vi "BuildMaun.vi"(8 "error in (no error)":errorcluster, 10 "menu reference":refnum<k9>, 11 "PLC_Module in":refnum<class "PLC_Module.lvclass">) -> (0 "error out":errorcluster, 3 "PLC_Module out":refnum<class "PLC_Module.lvclass">)   [LabVIEW 2025, in "PLC_Module.lvlib" / "PLC_Module.lvclass"]
uses:
  PLC_Module.lvclass
  PLC_Module.lvclass/PLC_Module.ctl
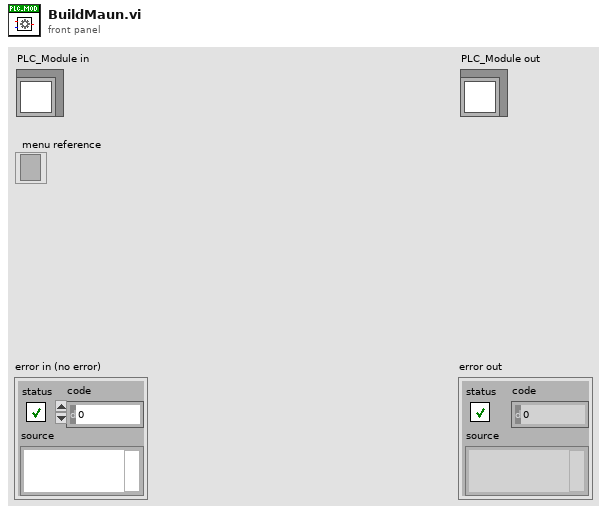
[diagram p1: front panel]
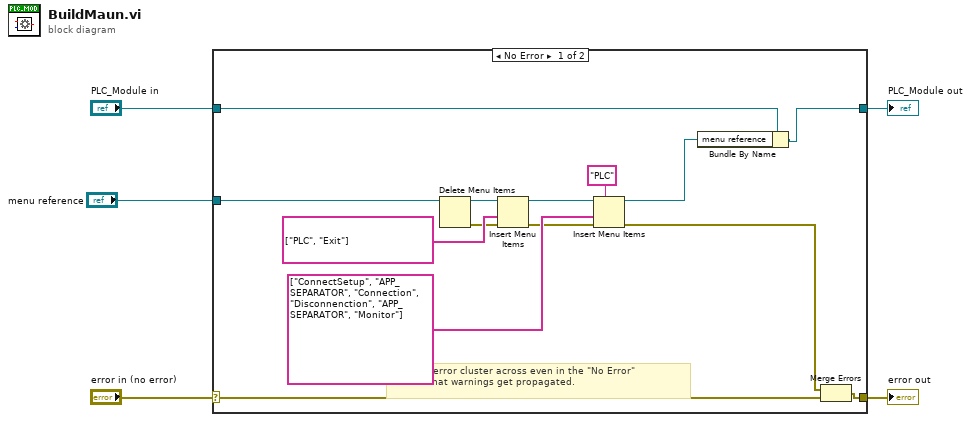
[diagram p0: block diagram]
diagram:
  n1 = case shown="No Error" "error in (no error)" {
    selector: "error in (no error)" -> [w19 w21]
    tunnel: [w13 w21] -> w4
    tunnel: [w6 w20] -> w2
    tunnel: "PLC_Module in" -> [w8 w20]
    tunnel: "menu reference" -> [w11 _]
    frame No Error {
      # "Wire the error cluster across even in the \"No Error\"\ncase so that warnings get propagated."
      n2 = Delete Menu Items(9:w11) -> (0:w9:errorcluster, 3:w10:refnum<k9>)  [unwired: 3 in]
      n3 = Insert Menu Items(6:w9, 7:string[] ["PLC", "Exit"] ("item tags"), 9:w10) -> (0:w14:errorcluster, 3:w17:refnum<k9>)  [unwired: 3 in, 1 out]
      n4 = Insert Menu Items(5:"PLC", 6:w14, 7:string[] ["ConnectSetup", "APP_SEPARATOR", "Connection", "Disconnenction", "APP_SEPARATOR", "Monitor"] ("item tags"), 9:w17) -> (0:w12:errorcluster, 3:w7:refnum<k9>)  [unwired: 2 in, 1 out]
      n5 = Bundle By Name(cluster=w8, "menu reference"=w7) -> (w6:refnum<class "PLC_Module.lvclass">)
      n6 = Merge Errors(w12, w19) -> (w13:errorcluster)
    }
    frame Error {
    }
  }
  "error out" <- w4
  "PLC_Module out" <- w2
